vi "Handle error.vi"(8 "error in (no error)":T1, 10 "module loopdata":T2) -> ()   [LabVIEW 2019, in "DataManagment.lvlib"]
uses:
  DataManagment.lvlib
  module data.ctl
  SubVIs/mmWave data_class/mmWave data.lvclass
  DM signal group.ctl
  SubVIs/Shared/Shared.lvlib
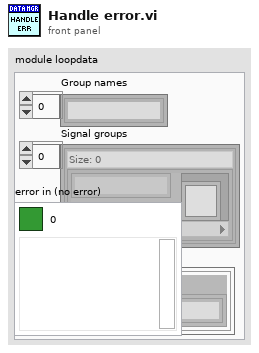
[diagram p1: front panel]
types:
  T1 = cluster{"Boolean Round":bool, "code":i32, "source":string}
  T2 = typedef "DataManagment.lvlib/module data.ctl" = cluster{"Group names":string[], "Signal groups":map{string, refnum<class "mmWave data.lvclass">}[], "groups":T3[]}
  T3 = typedef "DataManagment.lvlib/DM signal group.ctl" = cluster{"history":string[]}
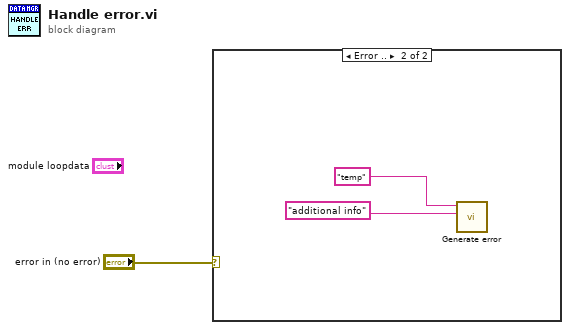
[diagram p0: block diagram]
diagram:
  n1 = case shown="Error .." "error in (no error)" {
    frame No Error {
    }
    frame Error {
      n2 = call "Generate error.vi"("info"="additional info" ("module"), "module"="temp") -> ()  [unwired: 9 in, 1 out]
    }
  }
